vi "Get Session and Channels (Poly).vi"   [LabVIEW 2020, in "Measurement Service Helpers.lvlib"]
doc: "Gets the session index and channel list for the sessions that correspond to the given pin name input. The session index can be used to access the given session information array."
uses:
  Measurement Service Helpers.lvlib
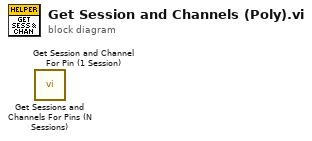
[diagram p0: block diagram]
diagram:
  n1 = call "Get Sessions and Channels For Pins (N Sessions).vi"() -> ()  [unwired: 9 in, 3 out]
  n2 = call "Get Session and Channel For Pin (1 Session).vi"() -> ()  [unwired: 9 in, 3 out]
